vi "Sprinkler.vi"() -> ()   [LabVIEW 2015]
uses:
  Boiler (100926F-01)/Solution/Controls/status.ctl
  Controls/data cluster.ctl
  Controls/timer status.ctl
panel:
  out "data cluster out":T1
  in  "time":dbl
  in  "data cluster":T1
  in  "direction":string
  out "error out":errorcluster
  in  "error in":errorcluster
  in  "Zone Setup Array":cluster{"Zone Selector":string, "Timing":dbl}[](array[cluster])
  out "Controller Status":string
  out "Zone Indicators":T2
  in  "Water Pressure Sensor (%)":u32(slide) scale=0.0..100.0
  in  "Rain Sensor":bool
  in  "Run Selector":bool
  in  "Setup":bool
  in  "Start":bool
  in  "stop":bool
  # "Controls"
  # "Simulation Controls"
  # "Rain"
  # "No Rain"
  # "Continuous"
  # "Single"
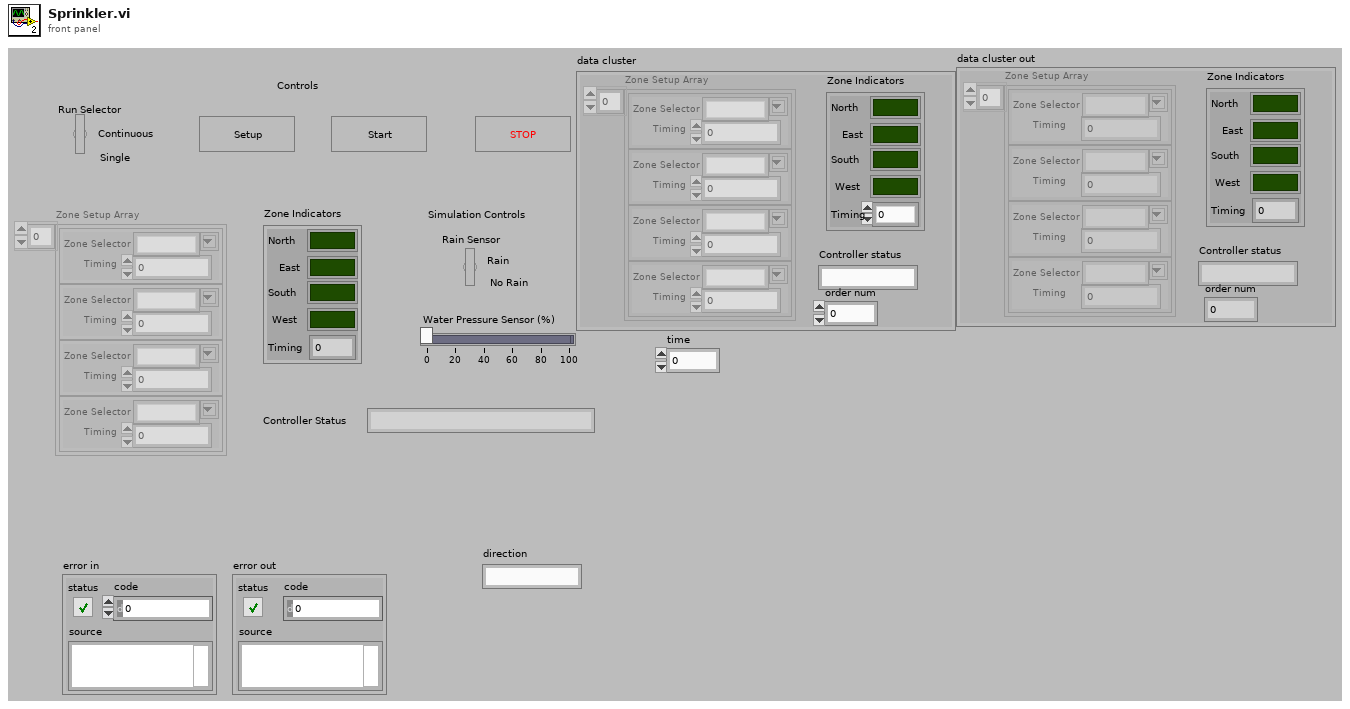
[diagram p1: front panel]
types:
  T1 = typedef "data cluster.ctl" = cluster{"Zone Setup Array":cluster{"Zone Selector":string, "Timing":dbl}[], "Zone Indicators":cluster{"North":bool, "East":bool, "South":bool, "West":bool, "Timing":u32}, "Controller status":string, "order num":i32}
  T2 = cluster{"North":bool, "East":bool, "South":bool, "West":bool, "Timing":u32}
  T3 = typedef "status.ctl" = enum16{"Error", "Setup", "Execute", "Exit", "Idle", "Initialize"}
  T4 = enum8{"Enabled", "Disabled", "Disabled and Grayed Out"}
  T5 = typedef "timer status.ctl" = enum16{"stop", "start"}
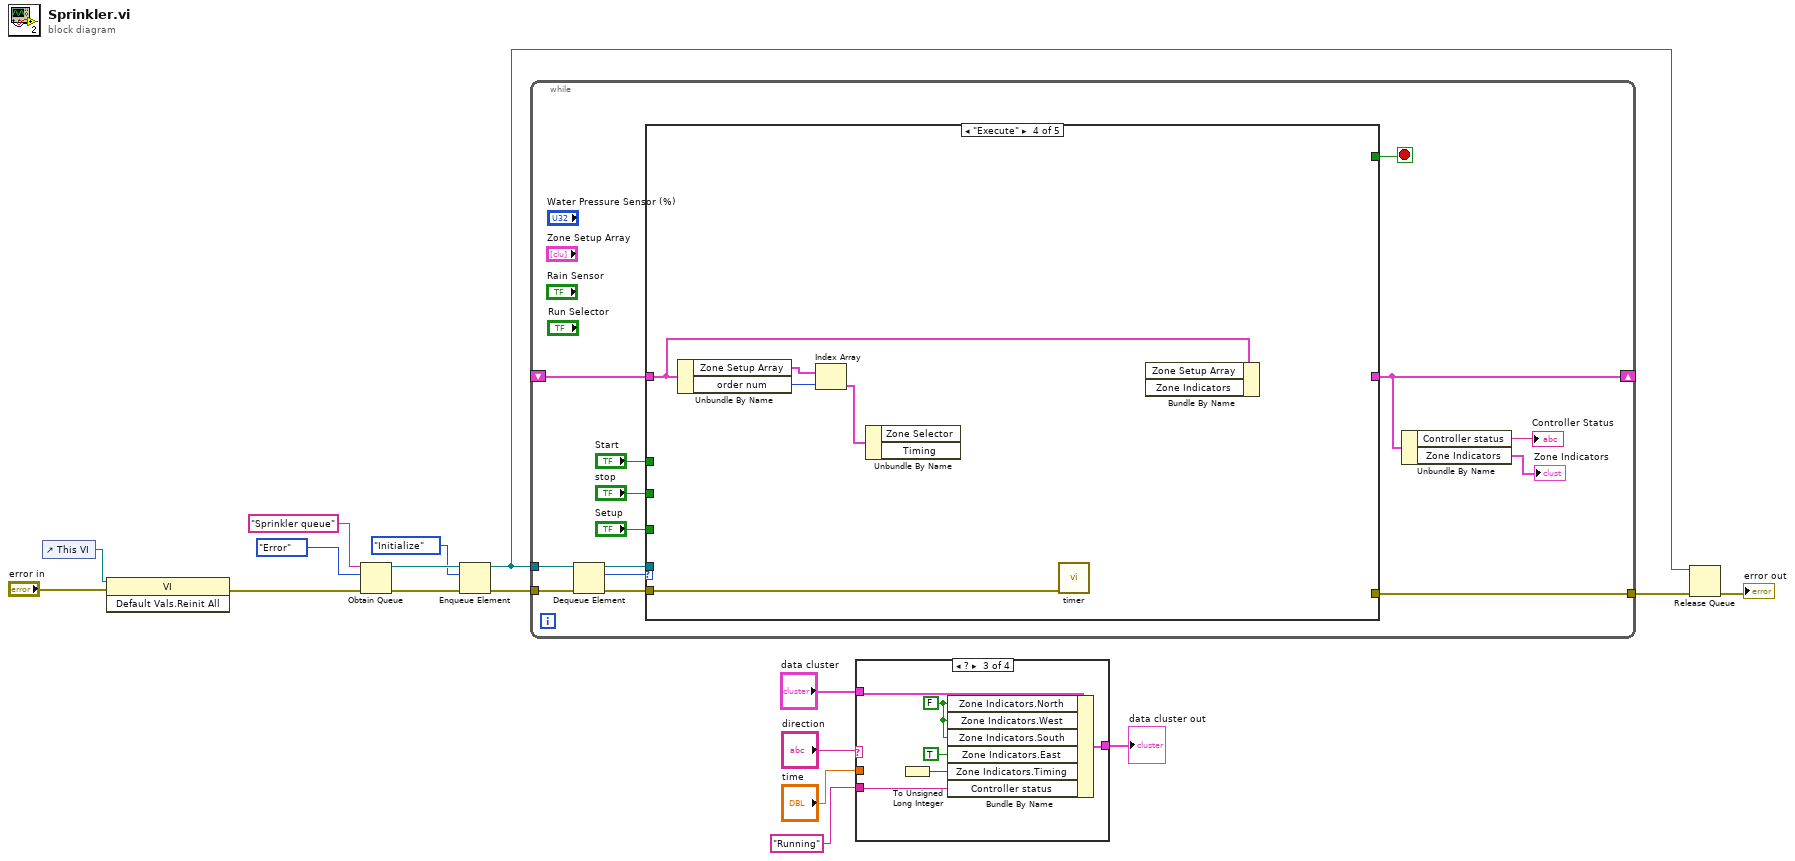
[diagram p0: block diagram]
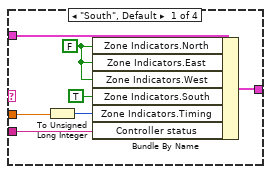
[diagram p2: hidden frame]
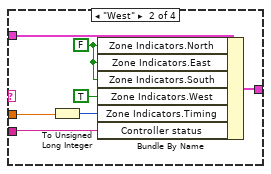
[diagram p3: hidden frame]
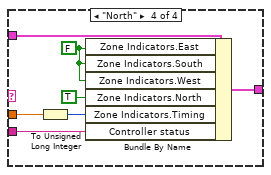
[diagram p4: hidden frame]
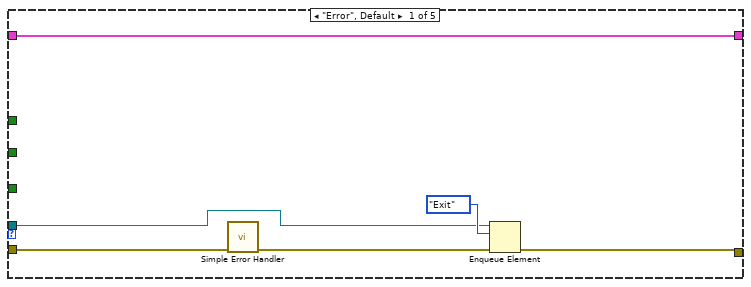
[diagram p5: hidden frame]
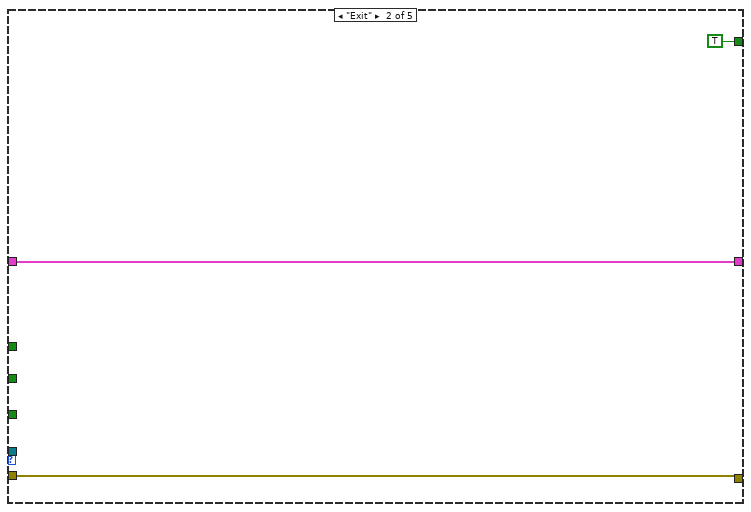
[diagram p6: hidden frame]
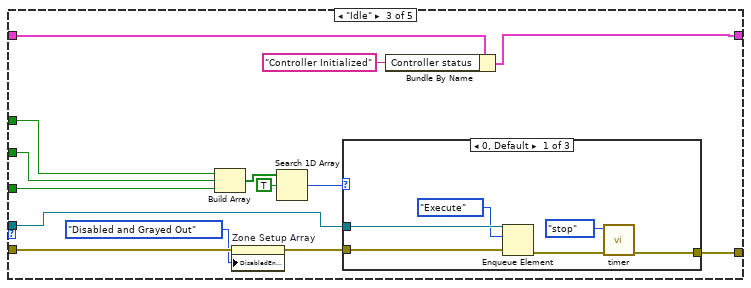
[diagram p7: hidden frame]
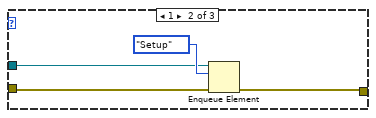
[diagram p8: hidden frame]
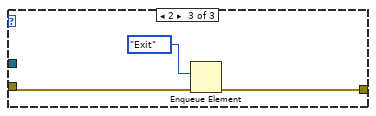
[diagram p9: hidden frame]
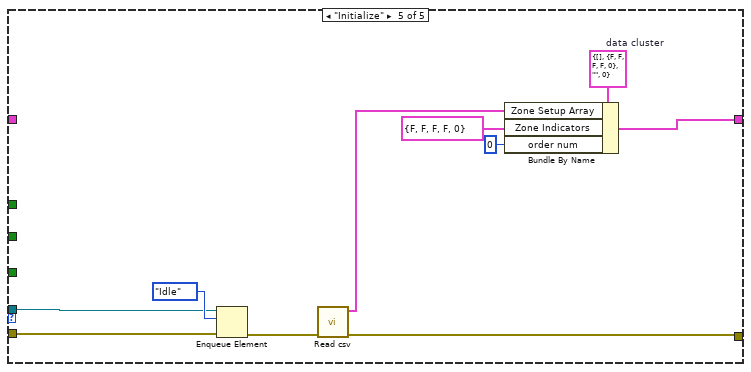
[diagram p10: hidden frame]
diagram:
  n1 = control-ref of="This VI"() -> (w8:refnum<vi>)
  n2 = invoke class="VI" method="Default Vals.Reinit All"(reference=w8, error in="error in") -> (error out=w6:errorcluster)  [unwired: 1 in, 2 out]
  n3 = Obtain Queue(name (unnamed)="Sprinkler queue", element data type=status."Error" ("status"), error in (no error)=w6) -> (queue out=w15:refnum<queue>, error out=w17:errorcluster)  [unwired: 2 in, 1 out]
  n4 = Enqueue Element(queue=w15, element=status."Initialize" ("status 2"), error in (no error)=w17) -> (queue out=w9:refnum<queue>, error out=w16:errorcluster)  [unwired: 1 in, 1 out]
  n5 = while {
    tunnel: w16 -> [w31]
    tunnel: w9 -> [w29]
    tunnel: [w26] -> w11
    shift-right: [w25] -> _
    shift-left: _ -> [w22]
    stop <- w21 stop-if-true
    n6 = Dequeue Element(queue=w29, error in (no error)=w31) -> (queue out=w27:refnum<queue>, element=w28:T3, error out=w30:errorcluster)  [unwired: 1 in, 1 out]
    n7 = case shown="\"Execute\"" w28 {
      tunnel: w30 -> [w35 w39 w54 w69 w81]
      tunnel: w27 -> [w32 _ w47 _ w80]
      tunnel: [w36 w39 w48 _ w78] -> w26
      tunnel: [w33 w38 w50 _ w74] -> w25
      tunnel: w22 -> [w33 w38 w52 w68 _]
      tunnel: [_ TRUE _ _ _] -> w21
      tunnel: "Setup" -> [_ _ w46 _ _]
      tunnel: "stop" -> [_ _ w45 _ _]
      tunnel: "Start" -> [_ _ w44 _ _]
      frame "Error", Default {
        n8 = call <vilib>:"Simple Error Handler.vi"("error in (no error)"=w35) -> ("error out"=w34:errorcluster)  [unwired: 4 in, 4 out]
        n9 = Enqueue Element(queue=w32, element=status."Exit" ("status 2"), error in (no error)=w34) -> (error out=w36:errorcluster)  [unwired: 1 in, 2 out]
      }
      frame "Exit" {
      }
      frame "Idle" {
        n10 = Build Array(w44, w45, w46) -> (w43:bool[])
        n11 = property on="Zone Setup Array" class="Arr (strict)"(error in=w54, "DisabledEnum"=T4."Disabled and Grayed Out" ("Disabled")) -> (error out=w49:errorcluster)  [unwired: 1 in, 1 out]
        n12 = Search 1D Array(1D array=w43, element=TRUE) -> (index of element=w41:i32)  [unwired: 1 in]
        n13 = case shown="0, Default" w41 {
          tunnel: w49 -> [w59 w63 w66]
          tunnel: [w56 w62 w65] -> w48
          tunnel: w47 -> [w60 w61 _]
          frame 0, Default {
            n14 = Enqueue Element(queue=w60, element=status."Execute" ("status 2"), error in (no error)=w59) -> (error out=w57:errorcluster)  [unwired: 1 in, 2 out]
            n15 = call "timer.vi"("error in"=w57, "timer status"=timer_status."stop") -> ("error out"=w56:errorcluster)  [unwired: 7 in, 2 out]
          }
          frame 1 {
            n16 = Enqueue Element(queue=w61, element=status."Setup" ("status 2"), error in (no error)=w63) -> (error out=w62:errorcluster)  [unwired: 1 in, 2 out]
          }
          frame 2 {
            n17 = Enqueue Element(element=status."Exit" ("status 2"), error in (no error)=w66) -> (error out=w65:errorcluster)  [unwired: 2 in, 2 out]
          }
        }
        n18 = Bundle By Name(cluster=w52, "Controller status"="Controller Initialized") -> (w50:T1)
      }
      frame "Execute" {
        n19 = Unbundle By Name(w68) -> ("Zone Setup Array"=w71:cluster{"Zone Selector":string, "Timing":dbl}[], "order num"=w72:i32)
        n20 = Index Array(array=w71, index=w72) -> (element=w70:cluster{"Zone Selector":string, "Timing":dbl})
        n21 = Unbundle By Name(w70) -> ()  [unwired: 2 out]
        n22 = call "timer.vi"("error in"=w69) -> ()  [unwired: 8 in, 3 out]
        n23 = Bundle By Name(cluster=w68) -> ()  [unwired: 2 in, 1 out]
      }
      frame "Initialize" {
        w77 = T1 {"Zone Setup Array"=[], "Zone Indicators"={"North"=FALSE, "East"=FALSE, "South"=FALSE, "West"=FALSE, "Timing"=0}, "Controller status"="", "order num"=0}  # data cluster
        n24 = Enqueue Element(queue=w80, element=status."Idle" ("status 2"), error in (no error)=w81) -> (error out=w79:errorcluster)  [unwired: 1 in, 2 out]
        n25 = call "Read csv.vi"("error in (no error)"=w79) -> ("error out"=w78:errorcluster, "Zone Setup"=w76:cluster{"Zone Selector":string, "Timing":dbl}[])  [unwired: 9 in]
        n26 = Bundle By Name(cluster=w77, "Zone Setup Array"=w76, "Zone Indicators"=T2 {"North"=FALSE, "East"=FALSE, "South"=FALSE, "West"=FALSE, "Timing"=0}, "order num"=0) -> (w74:T1)
      }
    }
    n27 = Unbundle By Name(w25) -> ("Controller status"=→"Controller Status":string, "Zone Indicators"=→"Zone Indicators":T2)
  }
  n28 = case "direction" {
    tunnel: "data cluster" -> [w85 w92 w98 w109]
    tunnel: "time" -> [w86 w91 _ w106]
    tunnel: "Running" ("Controller status") -> [w87 w94 w97 w105]
    tunnel: [w84 w93 w99 w104] -> w1
    frame "South", Default {
      w83 = FALSE ("Zone Indicators.North")
      n29 = To Unsigned Long Integer(number=w86) -> (unsigned 32bit integer=w89:u32)
      n30 = Bundle By Name(cluster=w85, "Zone Indicators.North"=w83, "Zone Indicators.East"=w83, "Zone Indicators.West"=w83, "Zone Indicators.South"=TRUE ("Zone Indicators.North"), "Zone Indicators.Timing"=w89, "Controller status"=w87) -> (w84:T1)
    }
    frame "West" {
      w90 = FALSE ("Zone Indicators.North")
      n31 = To Unsigned Long Integer(number=w91) -> (unsigned 32bit integer=w95:u32)
      n32 = Bundle By Name(cluster=w92, "Zone Indicators.North"=w90, "Zone Indicators.East"=w90, "Zone Indicators.South"=w90, "Zone Indicators.West"=TRUE ("Zone Indicators.North"), "Zone Indicators.Timing"=w95, "Controller status"=w94) -> (w93:T1)
    }
    frame ? {
      w102 = FALSE ("Zone Indicators.North")
      n33 = To Unsigned Long Integer() -> (unsigned 32bit integer=w101:u32)  [unwired: 1 in]
      n34 = Bundle By Name(cluster=w98, "Zone Indicators.North"=w102, "Zone Indicators.West"=w102, "Zone Indicators.South"=w102, "Zone Indicators.East"=TRUE ("Zone Indicators.North"), "Zone Indicators.Timing"=w101, "Controller status"=w97) -> (w99:T1)
    }
    frame "North" {
      w103 = FALSE ("Zone Indicators.North")
      n35 = To Unsigned Long Integer(number=w106) -> (unsigned 32bit integer=w108:u32)
      n36 = Bundle By Name(cluster=w109, "Zone Indicators.East"=w103, "Zone Indicators.South"=w103, "Zone Indicators.West"=w103, "Zone Indicators.North"=TRUE, "Zone Indicators.Timing"=w108, "Controller status"=w105) -> (w104:T1)
    }
  }
  "data cluster out" <- w1
  n37 = Release Queue(queue=w9, error in (no error)=w11) -> (error out=→"error out":errorcluster)  [unwired: 1 in, 2 out]
